vi "PlotVoxel.vi"(4 "Update time":dbl, 5 "Map Data In":T2(array[cluster]), 6 "Sensor position":cluster{"X":sgl, "Y":sgl, "Z":sgl}={"X"=0.0, "Y"=0.0, "Z"=70.75}, 7 "Chunk length":u8=8, 8 "voxel length":dbl=8.0 format="%#_13g", 9 "Window Bounds":T1={"Left"=0, "Top"=0, "Right"=750, "Bottom"=750}) -> ()   [LabVIEW 2014]
uses:
  <vilib>/Utility/miscctls.llb/LVRectTypeDef.ctl
  <vilib>/Utility/miscctls.llb/LV3DPointTypeDef.ctl
  <vilib>/picture/3D Picture Control/Object/Create Object (name).vi
  <vilib>/picture/3D Picture Control/Helpers/Set Light (no reference).vi
  <vilib>/picture/3D Picture Control/NI_3D Picture Control.lvlib
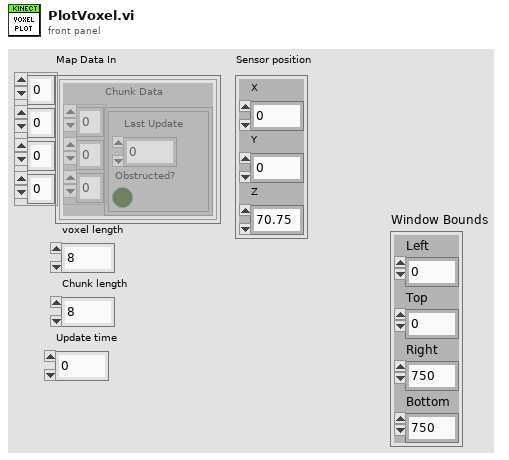
[diagram p1: front panel]
types:
  T1 = typedef "LVRectTypeDef.ctl" = cluster{"Left":i16, "Top":i16, "Right":i16, "Bottom":i16}
  T2 = cluster{"Chunk Data":cluster{"Last Update":u32, "Obstructed?":bool}[][][]}[][][][]
  T3 = typedef "LV3DPointTypeDef.ctl" = cluster{"X":sgl, "Y":sgl, "Z":sgl}
  T4 = cluster{"Base Height":sgl, "Base Height":sgl, "element":dbl}
  T5 = enum16{"Inherit Value", "Points", "Wireframe", "Polygons"}
  T6 = cluster{"Chunk Data":cluster{"Last Update":u32, "Obstructed?":bool}[][][]}
  T7 = cluster{"Last Update":u32, "Obstructed?":bool}[][][]
  T8 = enum16{"Open", "Minimized", "Maximized", "Hidden"}
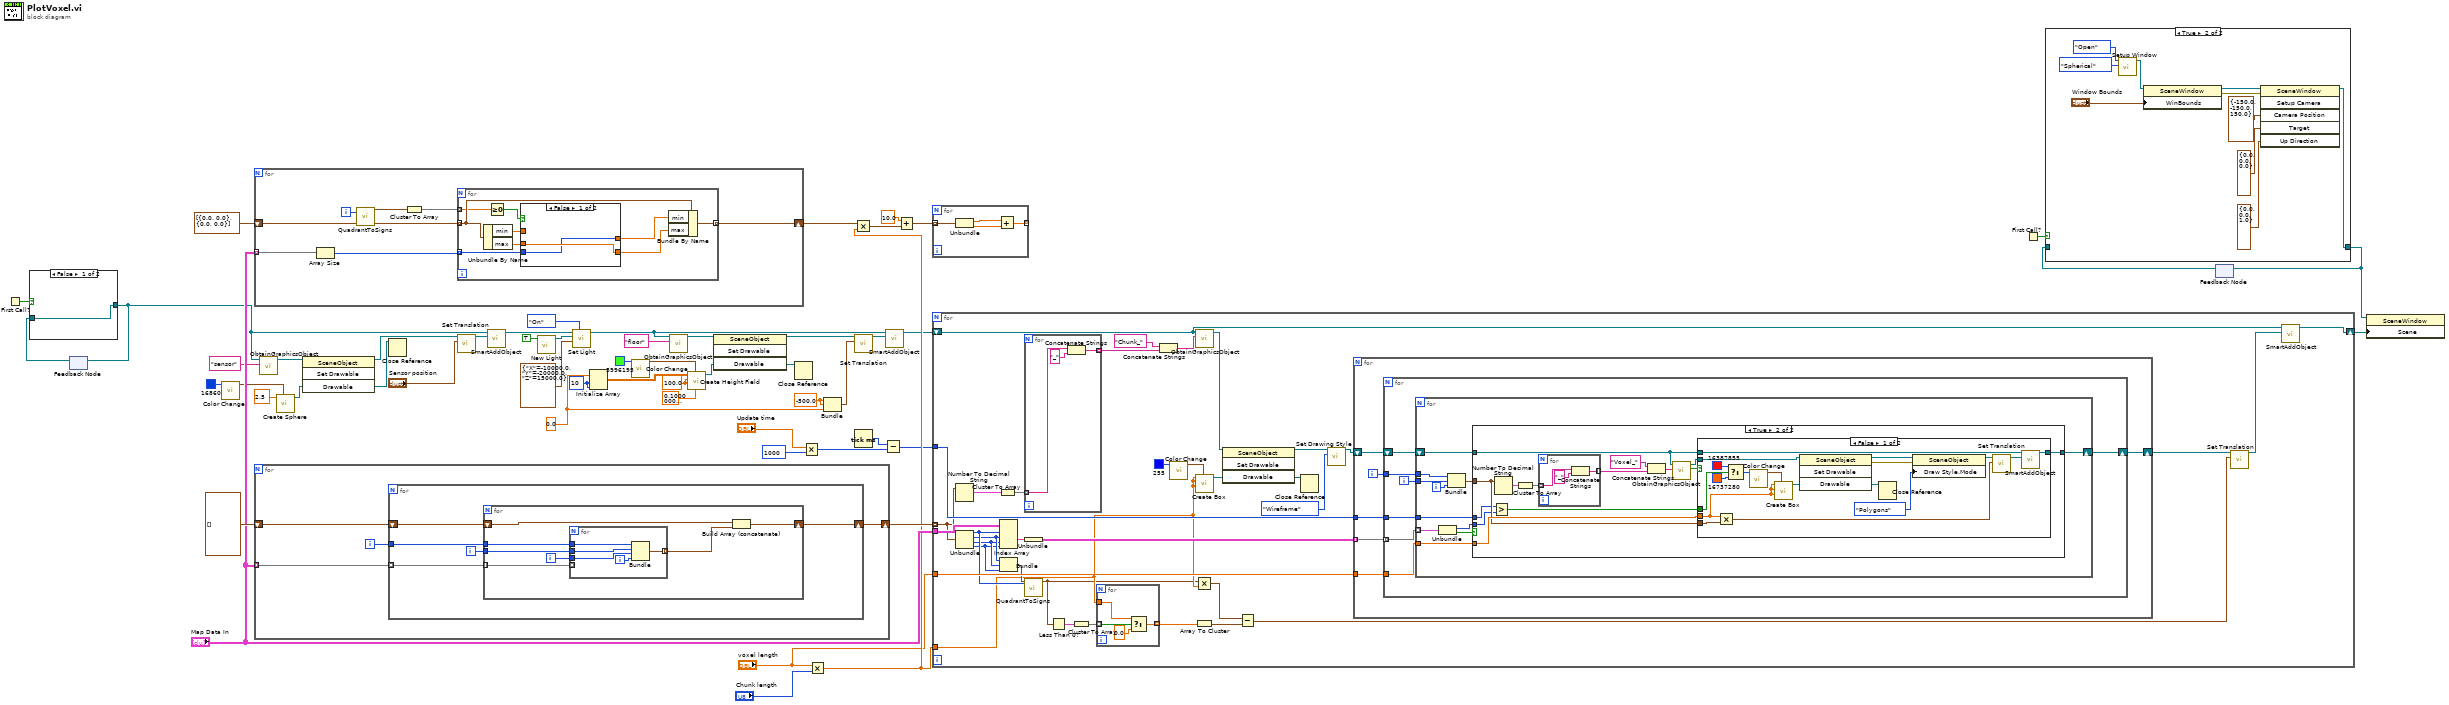
[diagram p0: block diagram]
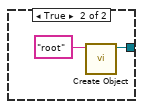
[diagram p2: hidden frame]
diagram:
  w24 = sgl 100.0 ("Row Interval")
  w25 = 10 ("dimension size")
  w27 = sgl -500.0 ("Base Height")
  w30 = 0.0 ("element")
  n1 = First Call?() -> (First Call?: T/F=w1:bool)
  n2 = feedback #1() -> (w2:refnum<vi>)  [unwired: 1 in]
  n3 = case shown="False" w1 {
    tunnel: [w56 w57] -> w3
    tunnel: w2 -> [w56 _]
    frame False {
    }
    frame True {
      n4 = call-poly <vilib>:"Create Object.vi"("Name"="root") -> ("Scene:New Object"=w57:refnum<vi>)  [unwired: 9 in, 1 out]
    }
  }
  n5 = feedback-in #1(w3) -> ()
  n6 = call <vilib>:"Color Change.vi"("Color"=u32 16860) -> ("RGBA"=w16:cluster{"R":sgl, "G":sgl, "B":sgl, "A":sgl})  [unwired: 10 in]
  n7 = for {
    tunnel: "Map Data In" -> [w64] mode=indexing
    shift-right: [w59] -> w50
    shift-left: cluster{"min":dbl, "max":dbl}[] [{"min"=0.0, "max"=0.0}, {"min"=0.0, "max"=0.0}] -> [w63]
    i -> [w65]
    n8 = Array Size(array=w64) -> (size(s)=w62:i32[])
    n9 = call "QuadrantToSigns.vi"("Quadrant"=w65) -> ("Point Out"=w61:cluster{"X":sgl, "Y":sgl, "Z":sgl})  [unwired: 18 in]
    n10 = Cluster To Array(cluster=w61) -> (array=w60:sgl[])
    n11 = for {
      tunnel: w63 -> [w73] mode=indexing
      tunnel: w62 -> [w68] mode=indexing
      tunnel: w60 -> [w67] mode=indexing
      tunnel: [w74] -> w59 mode=indexing
      n12 = Unbundle By Name(w73) -> ("min"=w72:dbl, "max"=w71:dbl)
      n13 = Greater Or Equal To 0?(x=w67) -> (x >= 0?=w66:bool)
      n14 = case shown="False" w66 {
        tunnel: w68 -> [w75 w77]
        tunnel: w72 -> [_ w78]
        tunnel: w71 -> [w76 _]
        tunnel: [w75 w78] -> w70
        tunnel: [w76 w77] -> w69
        frame False {
        }
        frame True {
        }
      }
      n15 = Bundle By Name(cluster=w73, "min"=w70, "max"=w69) -> (w74:cluster{"min":dbl, "max":dbl})
    }
  }
  n16 = for {
    tunnel: "Map Data In" -> [w79] mode=indexing
    shift-right: [w81] -> w40
    shift-left: cluster{i32, i32, i32, i32}[] [] -> [w80]
    i -> [w82]
    n17 = for {
      tunnel: w79 -> [w87] mode=indexing
      tunnel: w82 -> [w86]
      shift-right: [w84] -> w81
      shift-left: w80 -> [w83]
      i -> [w85]
      n18 = for {
        tunnel: w87 -> [w94] mode=indexing
        tunnel: w86 -> [w93]
        tunnel: w85 -> [w92]
        shift-right: [w90] -> w84
        shift-left: w83 -> [w89]
        i -> [w91]
        n19 = for {
          tunnel: w94 -> [_] mode=indexing
          tunnel: w93 -> [w99]
          tunnel: w92 -> [w98]
          tunnel: w91 -> [w97]
          tunnel: [w95] -> w88 mode=indexing
          i -> [w96]
          n20 = Bundle(w99, w98, w97, w96) -> (w95:cluster{i32, i32, i32, i32})  [unwired: 1 in]
        }
        n21 = Build Array (concatenate)(w89, w88) -> (w90:cluster{i32, i32, i32, i32}[])
      }
    }
  }
  n22 = call "ObtainGraphicsObject.vi"("Object Name"="sensor" ("Name"), "Scene in"=w3) -> ("Scene:New Object"=w14:refnum<vi>)  [unwired: 8 in, 1 out]
  n23 = call <vilib>:"Create Sphere.vi"("Color"=w16, "Radius"=sgl 2.5) -> ("New Sphere Refnum"=w13:refnum<vi>)  [unwired: 8 in, 1 out]
  n24 = invoke class="SceneObject" method="Set Drawable"(reference=w14, "Drawable"=w13) -> (reference out=w11:refnum<vi>, "Drawable"=w12:refnum<vi>)  [unwired: 2 in, 2 out]
  n25 = Close Reference(reference=w12) -> ()  [unwired: 1 in, 1 out]
  n26 = call <vilib>:"Set Translation.vi"("Translation"="Sensor position", "Scene Object"=w11) -> ("Translated Object"=w9:refnum<vi>)  [unwired: 8 in, 1 out]
  n27 = call "SmartAddObject.vi"("New Object In"=w9, "Scene Object In"=w3) -> ("Scene Object Out"=w8:refnum<vi>)  [unwired: 8 in, 1 out]
  n28 = call <vilib>:"New Light.vi"("At Infinity"=TRUE) -> ("New Light Refnum"=w21:refnum<vi>)  [unwired: 9 in, 1 out]
  n29 = call-poly <vilib>:"Set Light.vi"("Light State"=enum16{"Inherit Value", "Off", "On"}."On", "Position"=T3 {"X"=-10000.0, "Y"=-20000.0, "Z"=15000.0}, "Light Refnum In"=w21, "Scene Object In"=w8) -> ("Scene Object Out"=w22:refnum<vi>)  [unwired: 6 in, 1 out]
  n30 = Initialize Array(w30, w25, w25) -> (w46:dbl[][])
  n31 = call <vilib>:"Color Change.vi"("Color"=u32 3996195) -> ("RGBA"=w54:cluster{"R":sgl, "G":sgl, "B":sgl, "A":sgl})  [unwired: 10 in]
  n32 = call "ObtainGraphicsObject.vi"("Object Name"="floor" ("Name"), "Scene in"=w22) -> ("Scene:New Object"=w43:refnum<vi>)  [unwired: 8 in, 1 out]
  n33 = call <vilib>:"Create Height Field.vi"("Base Height"=sgl 0.1, "Color"=w54, "Column Interval"=w24, "Row Interval"=w24, "Data"=w46) -> ("New Height Field Refnum"=w52:refnum<vi>)  [unwired: 5 in, 1 out]
  n34 = invoke class="SceneObject" method="Set Drawable"(reference=w43, "Drawable"=w52) -> (reference out=w41:refnum<vi>, "Drawable"=w45:refnum<vi>)  [unwired: 2 in, 2 out]
  n35 = Close Reference(reference=w45) -> ()  [unwired: 1 in, 1 out]
  n36 = Multiply(x="Update time", y=u32 1000) -> (x*y=w34:u32)
  n37 = Multiply(x="voxel length", y="Chunk length") -> (x*y=w38:dbl)
  n38 = Bundle("Base Height"=w27, "Base Height"=w27, "element"=w30) -> (w26:T4)  [unwired: 1 in]
  n39 = Multiply(x=w50, y=w38) -> (x*y=w48:cluster{"min":dbl, "max":dbl}[])
  n40 = call <vilib>:"Set Translation.vi"("Translation"=w26, "Scene Object"=w41) -> ("Translated Object"=w28:refnum<vi>)  [unwired: 8 in, 1 out]
  n41 = Tick Count (ms)() -> (millisecond timer value=w35:u32)
  n42 = Subtract(x=w35, y=w34) -> (x-y=w33:u32)
  n43 = call "SmartAddObject.vi"("New Object In"=w28, "Scene Object In"=w22) -> ("Scene Object Out"=w29:refnum<vi>)  [unwired: 8 in, 1 out]
  n44 = Add(x=10.0, y=w48) -> (x+y=w47:cluster{"min":dbl, "max":dbl}[])
  n45 = for {
    tunnel: w47 -> [w103] mode=indexing
    tunnel: [w101] -> _ mode=indexing
    n46 = Unbundle(w103) -> ("min"=w100:dbl, "max"=w102:dbl)
    n47 = Add(x=w100, y=w102) -> (x+y=w101:dbl)
  }
  n48 = for {
    tunnel: w40 -> [w110] mode=indexing
    shift-right: [w112] -> w7
    shift-left: w29 -> [w113]
    tunnel: w38 -> [w106]
    tunnel: "Map Data In" -> [w132]
    tunnel: w33 -> [w127]
    tunnel: "voxel length" -> [w126]
    n49 = Number To Decimal String(number=w110) -> (decimal integer string=w109:cluster{string, string, string, string})  [unwired: 1 in]
    n50 = Unbundle(w110) -> (w125:i32, w124:i32, w123:i32, w122:i32)
    n51 = Cluster To Array(cluster=w109) -> (array=w108:string[])
    n52 = Index Array(array=w132, index (dim 0)=w125, index (dim 1)=w124, index (dim 2)=w123, index (dim 3)=w122) -> (element=w131:T6)
    n53 = Bundle(w124, w123, w122) -> (w121:cluster{i32, i32, i32})  [unwired: 1 in]
    n54 = for {
      tunnel: w108 -> [w142] mode=indexing
      tunnel: [w140] -> w107 mode=indexing
      n55 = Concatenate Strings(w142, "_" ("element")) -> (w140:string)
    }
    n56 = Unbundle(w131) -> ("Chunk Data"=w128:T7)
    n57 = call "QuadrantToSigns.vi"("Point"=w121, "Quadrant"=w125) -> ("Point Out"=w105:cluster{"X":sgl, "Y":sgl, "Z":sgl})  [unwired: 17 in]
    n58 = Less Than 0?(x=w105) -> (x < 0?=w120:cluster{"X":bool, "Y":bool, "Z":bool})
    n59 = Cluster To Array(cluster=w120) -> (array=w119:bool[])
    n60 = for {
      tunnel: w119 -> [w146] mode=indexing
      tunnel: w106 -> [w145]
      tunnel: [w143] -> w118 mode=indexing
      n61 = Select(t=w145, s=w146, f=0.0) -> (s? t:f=w143:dbl)
    }
    n62 = Concatenate Strings("Chunk_", w107) -> (w138:string)
    n63 = call <vilib>:"Color Change.vi"("Color"=u32 255) -> ("RGBA"=w137:cluster{"R":sgl, "G":sgl, "B":sgl, "A":sgl})  [unwired: 10 in]
    n64 = Multiply(x=w105, y=w106) -> (x*y=w104:cluster{"X":dbl, "Y":dbl, "Z":dbl})
    n65 = Array To Cluster(array=w118) -> (cluster=w117:cluster{"[0]":dbl, "[1]":dbl, "[2]":dbl})
    n66 = call "ObtainGraphicsObject.vi"("Object Name"=w138, "Scene in"=w113) -> ("Scene:New Object"=w135:refnum<vi>)  [unwired: 8 in, 1 out]
    n67 = call <vilib>:"Create Box.vi"("Color"=w137, "Length Z"=w106, "Length Y"=w106, "Length X"=w106) -> ("New Box Refnum"=w134:refnum<vi>)  [unwired: 6 in, 1 out]
    n68 = invoke class="SceneObject" method="Set Drawable"(reference=w135, "Drawable"=w134) -> (reference out=w130:refnum<vi>, "Drawable"=w133:refnum<vi>)  [unwired: 2 in, 2 out]
    n69 = Subtract(x=w104, y=w117) -> (x-y=w114:cluster{dbl, dbl, dbl})
    n70 = Close Reference(reference=w133) -> ()  [unwired: 1 in, 1 out]
    n71 = call <vilib>:"Set Drawing Style.vi"("Mode"=T5."Wireframe", "Scene Object In"=w130) -> ("Scene Object Out"=w116:refnum<vi>)  [unwired: 8 in, 1 out]
    n72 = for {
      tunnel: w128 -> [w152] mode=indexing
      tunnel: w127 -> [w151]
      tunnel: w126 -> [w149]
      shift-right: [w147] -> w115
      shift-left: w116 -> [w148]
      i -> [w150]
      n73 = for {
        tunnel: w152 -> [w159] mode=indexing
        tunnel: w151 -> [w158]
        tunnel: w150 -> [w157]
        tunnel: w149 -> [w155]
        shift-right: [w153] -> w147
        shift-left: w148 -> [w154]
        i -> [w156]
        n74 = for {
          tunnel: w159 -> [w170] mode=indexing
          tunnel: w158 -> [w168]
          tunnel: w157 -> [w166]
          tunnel: w156 -> [w165]
          tunnel: w155 -> [w162]
          shift-right: [w160] -> w153
          shift-left: w154 -> [w161]
          i -> [w164]
          n75 = Unbundle(w170) -> ("Last Update"=w167:u32, "Obstructed?"=w169:bool)
          n76 = Bundle(w166, w165, w164) -> (w163:cluster{i32, i32, i32})  [unwired: 1 in]
          n77 = case shown="True" w169 {
            tunnel: w168 -> [_ w173]
            tunnel: w167 -> [_ w174]
            tunnel: w163 -> [_ w180]
            tunnel: w162 -> [_ w183]
            tunnel: w161 -> [w171 w182]
            tunnel: [w171 w181] -> w160
            frame False {
            }
            frame True {
              n78 = Greater?(x=w173, y=w174) -> (0:w172:bool)
              n79 = Number To Decimal String(number=w180) -> (decimal integer string=w179:cluster{string, string, string})  [unwired: 1 in]
              n80 = Cluster To Array(cluster=w179) -> (array=w176:string[])
              n81 = for {
                tunnel: w176 -> [w188] mode=indexing
                tunnel: [w186] -> w175 mode=indexing
                n82 = Concatenate Strings(w188, "_" ("element")) -> (w186:string)
              }
              n83 = Concatenate Strings("Voxel_", w175) -> (w184:string)
              n84 = call "ObtainGraphicsObject.vi"("Object Name"=w184, "Scene in"=w182) -> ("Found?"=w177:bool, "Scene:New Object"=w178:refnum<vi>)  [unwired: 8 in]
              n85 = case shown="False" w177 {
                tunnel: w183 -> [w203 _]
                tunnel: w182 -> [w201 w207]
                tunnel: [w199 w207] -> w181
                tunnel: w180 -> [w194 _]
                tunnel: w178 -> [w193 _]
                tunnel: w172 -> [w190 _]
                frame False {
                  n86 = Multiply(x=w203, y=w194) -> (x*y=w202:cluster{dbl, dbl, dbl})
                  n87 = Select(t=u32 16387855 ("Color"), s=w190, f=u32 16737280 ("Color")) -> (s? t:f=w192:u32)
                  n88 = call <vilib>:"Color Change.vi"("Color"=w192) -> ("RGBA"=w206:cluster{"R":sgl, "G":sgl, "B":sgl, "A":sgl})  [unwired: 10 in]
                  n89 = call <vilib>:"Create Box.vi"("Color"=w206, "Length Z"=w203, "Length Y"=w203, "Length X"=w203) -> ("New Box Refnum"=w205:refnum<vi>)  [unwired: 6 in, 1 out]
                  n90 = invoke class="SceneObject" method="Set Drawable"(reference=w193, "Drawable"=w205) -> (reference out=w198:refnum<vi>, error out=w197:errorcluster, "Drawable"=w204:refnum<vi>)  [unwired: 2 in, 1 out]
                  n91 = Close Reference(reference=w204) -> ()  [unwired: 1 in, 1 out]
                  n92 = property class="SceneObject"(reference=w198, error in=w197, "Draw Style.Mode"=T5."Polygons" ("Draw Style:Mode")) -> (reference out=w195:refnum<vi>)  [unwired: 1 out]
                  n93 = call <vilib>:"Set Translation.vi"("Translation"=w202, "Scene Object"=w195) -> ("Translated Object"=w200:refnum<vi>)  [unwired: 8 in, 1 out]
                  n94 = call "SmartAddObject.vi"("New Object In"=w200, "Scene Object In"=w201) -> ("Scene Object Out"=w199:refnum<vi>)  [unwired: 8 in, 1 out]
                }
                frame True {
                }
              }
            }
          }
        }
      }
    }
    n95 = call <vilib>:"Set Translation.vi"("Translation"=w114, "Scene Object"=w115) -> ("Translated Object"=w111:refnum<vi>)  [unwired: 8 in, 1 out]
    n96 = call "SmartAddObject.vi"("New Object In"=w111, "Scene Object In"=w113) -> ("Scene Object Out"=w112:refnum<vi>)  [unwired: 8 in, 1 out]
  }
  n97 = First Call?() -> (First Call?: T/F=w4:bool)
  n98 = feedback #2() -> (w5:refnum<vi>)  [unwired: 1 in]
  n99 = case shown="True" w4 {
    tunnel: [w208 w209] -> w6
    tunnel: w5 -> [w208 _]
    frame False {
    }
    frame True {
      n100 = call <vilib>:"Setup Window.vi"("Camera Controller"=enum16{"None", "Spherical", "Flying"}."Spherical", "Window State"=T8."Open") -> ("New Window Refnum"=w216:refnum<vi>)  [unwired: 8 in, 1 out]
      n101 = property class="SceneWindow"(reference=w216, "WinBounds"="Window Bounds") -> (reference out=w214:refnum<vi>, error out=w213:errorcluster)  [unwired: 1 in]
      n102 = invoke class="SceneWindow" method="Setup Camera"(reference=w214, error in=w213, "Camera Position"=T3 {"X"=-150.0, "Y"=-150.0, "Z"=150.0}, "Target"=T3 {"X"=0.0, "Y"=0.0, "Z"=0.0} ("Up Direction"), "Up Direction"=T3 {"X"=0.0, "Y"=0.0, "Z"=1.0}) -> (reference out=w209:refnum<vi>)  [unwired: 1 in, 5 out]
    }
  }
  n103 = feedback-in #2(w6) -> ()
  n104 = property class="SceneWindow"(reference=w6, "Scene"=w7) -> ()  [unwired: 1 in, 2 out]
